vi "Simulation Call Statechart (DLL).vi"(4 "operation":T6, 5 "Robot Index":i32, 8 "error in (no error)":errorcluster, 10 "Array Sensors In":T1[](array[typedef]) {"Kobuki Sensors"."Charger Source" items=["DISCHARGING"=0, "DOCKING_CHARGED"=2, "DOCKING_CHARGING"=6, "ADAPTER_CHARGED"=18, "ADAPTER_CHARGING"=22]; "accelerometer"."z axis (g)" format="%.3f"; "accelerometer"."y axis (g)" format="%.3f"; "accelerometer"."x axis (g)" format="%.3f"}, 11 "simulator":T7={"configuration"={"maxTime"=5.0, "enableVisualization"=TRUE, "Environment Definition"=path "simulation configuration.ini", "Record Location"=path "Simulation Record.xml", "autograde?"=TRUE, "interactive?"=FALSE, "Feedback Mode"=enum."debug navigation", "Robot State Charts"=[path "C:/Users/blueuser/Desktop/Robo Sim Berkley/cpsgrader-release-0.4/Simulators/EECS149lab/src/LabVIEW/statechart/Simulation Statechart.vi"], "statechart"=path "C:/Users/blueuser/Desktop/Robo Sim Berkley/cpsgrader-release-0.4/Simulators/EECS149lab/src/LabVIEW/statechart/Simulation Statechart.vi"}, "Statechart\ndisplay"=refnum, "first step?"=FALSE, "Robots Simulation Statecharts"=[], "Robots"=[]}) -> (0 "error out":errorcluster, 2 "Array Sensors Out":T1[](array[typedef]) {"Kobuki Sensors"."Charger Source" items=["DISCHARGING"=0, "DOCKING_CHARGED"=2, "DOCKING_CHARGING"=6, "ADAPTER_CHARGED"=18, "ADAPTER_CHARGING"=22]; "accelerometer"."z axis (g)" format="%.3f"; "accelerometer"."y axis (g)" format="%.3f"; "accelerometer"."x axis (g)" format="%.3f"}, 3 "simulator":T7={"configuration"={"maxTime"=5.0, "enableVisualization"=TRUE, "Environment Definition"=path "simulation configuration.ini", "Record Location"=path "Simulation Record.xml", "autograde?"=TRUE, "interactive?"=FALSE, "Feedback Mode"=enum."debug navigation", "Robot State Charts"=[path "C:/Users/blueuser/Desktop/Robo Sim Berkley/cpsgrader-release-0.4/Simulators/EECS149lab/src/LabVIEW/statechart/Simulation Statechart.vi"], "statechart"=path "C:/Users/blueuser/Desktop/Robo Sim Berkley/cpsgrader-release-0.4/Simulators/EECS149lab/src/LabVIEW/statechart/Simulation Statechart.vi"}, "Statechart\ndisplay"=refnum, "first step?"=FALSE, "Robots Simulation Statecharts"=[], "Robots"=[]})   [LabVIEW 2015]
uses:
  Simulator.ctl
  CyberSim interface/Simulation Configuration.ctl
  autograder/feedbackMode.ctl
  Multi Bot Code/RobotData.ctl
  <instrlib>/DC Motor Controller/HAIOL/DC Motor Controller.lvclass
  Simulation Call Statechart Operation.ctl
  shared/Sensors.ctl
  shared/Accelerometer.ctl
  Kobuki/KobukiSensors.ctl
  Kobuki/Kobuki Bumps and WheelDrops.ctl
  Kobuki/Kobuki Buttons.ctl
panel:
  # "Electrical: charging, battery, OI mode"
  # "Sensors: bump, cliff, button, wheel drop"
  # "Motors:"
  # "Inertia"
  # "Electrical: charging, battery, OI mode"
  # "Sensors: bump, cliff, button, wheel drop"
  # "Motors:"
  # "Inertia"
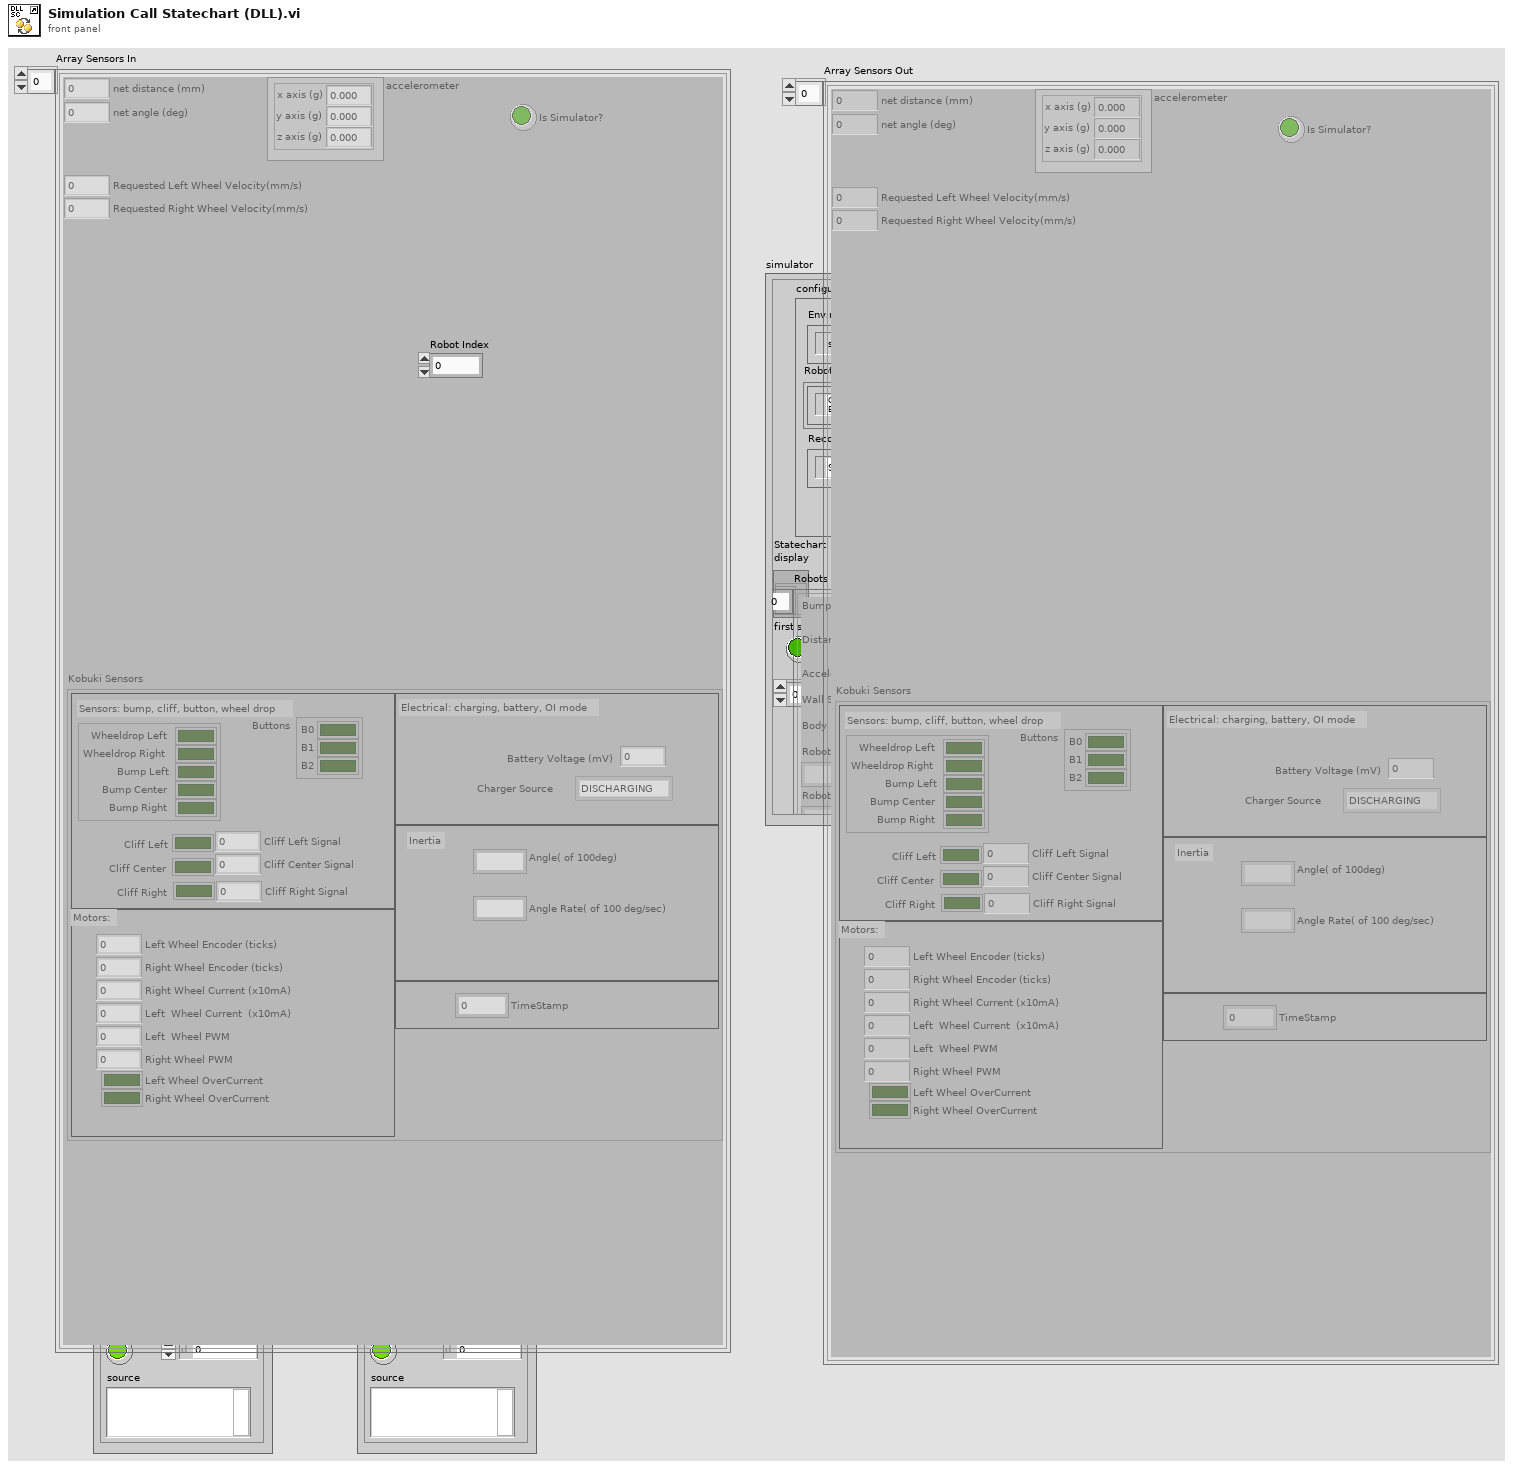
[diagram p1: front panel]
types:
  T1 = typedef "Sensors.ctl" = cluster{"net distance (mm)":i32, "net angle (deg)":i32, "accelerometer":T2, "Is Simulator?":bool, "Kobuki Sensors":T3, "Requested Left Wheel Velocity(mm/s)":i32, "Requested Right Wheel Velocity(mm/s)":i32}
  T2 = typedef "Accelerometer.ctl" = cluster{"x axis (g)":dbl, "y axis (g)":dbl, "z axis (g)":dbl}
  T3 = typedef "KobukiSensors.ctl" = cluster{"Bumps + Wheel Drops":T4, "Cliff Left":bool, "Cliff Center":bool, "Cliff Right":bool, "Cliff Left Signal":u16, "Cliff Center Signal":u16, "Cliff Right Signal":u16, "Buttons":T5, "Left Wheel Encoder (ticks)":u16, "Right Wheel Encoder (ticks) ":u16, "Left  Wheel PWM":i8, "Right Wheel PWM":i8, "Left Wheel OverCurrent":bool, "Right Wheel OverCurrent ":bool, "Right Wheel Current (x10mA)":i16, "Left  Wheel Current  (x10mA)":i16, "TimeStamp":u16, "Battery Voltage (mV)":i16, "Angle( of 100deg)":i16, "Angle Rate( of 100 deg/sec)":i16, "Charger Source ":i8}
  T4 = typedef "Kobuki Bumps and WheelDrops.ctl" = cluster{"Wheeldrop Left":bool, "Wheeldrop Right":bool, "Bump Left":bool, "Bump Center":bool, "Bump Right":bool}
  T5 = typedef "Kobuki Buttons.ctl" = cluster{"B0":bool, "B1":bool, "B2":bool}
  T6 = typedef "Simulation Call Statechart Operation.ctl" = enum16{"Initialize", "Call Statechart", "Finalize"}
  T7 = typedef "Simulator.ctl" = cluster{"configuration":T8, "Statechart\ndisplay":refnum<vi>, "first step?":bool, "Robots Simulation Statecharts":path[], "Robots":T10[]}
  T8 = typedef "Simulation Configuration.ctl" = cluster{"maxTime":sgl, "enableVisualization":bool, "Environment Definition":path, "Record Location":path, "autograde?":bool, "interactive?":bool, "Feedback Mode":T9, "Robot State Charts":path[], "statechart":path}
  T9 = typedef "feedbackMode.ctl" = enum32{"debug navigation", "debug hill climb", "autograde navigation", "autograde hill climb"}
  T10 = typedef "RobotData.ctl" = cluster{"Bump Sensors":refnum<k20>[], "Distance Sensors":refnum<k20>[], "Accelerometer":refnum<k20>, "Wall Sensor":refnum<k20>, "Body":refnum<k20>, "RobotID":string, "RobotType":string, "Left Motor":refnum<class "DC Motor Controller.lvclass">, "Right Motor":refnum<class "DC Motor Controller.lvclass">}
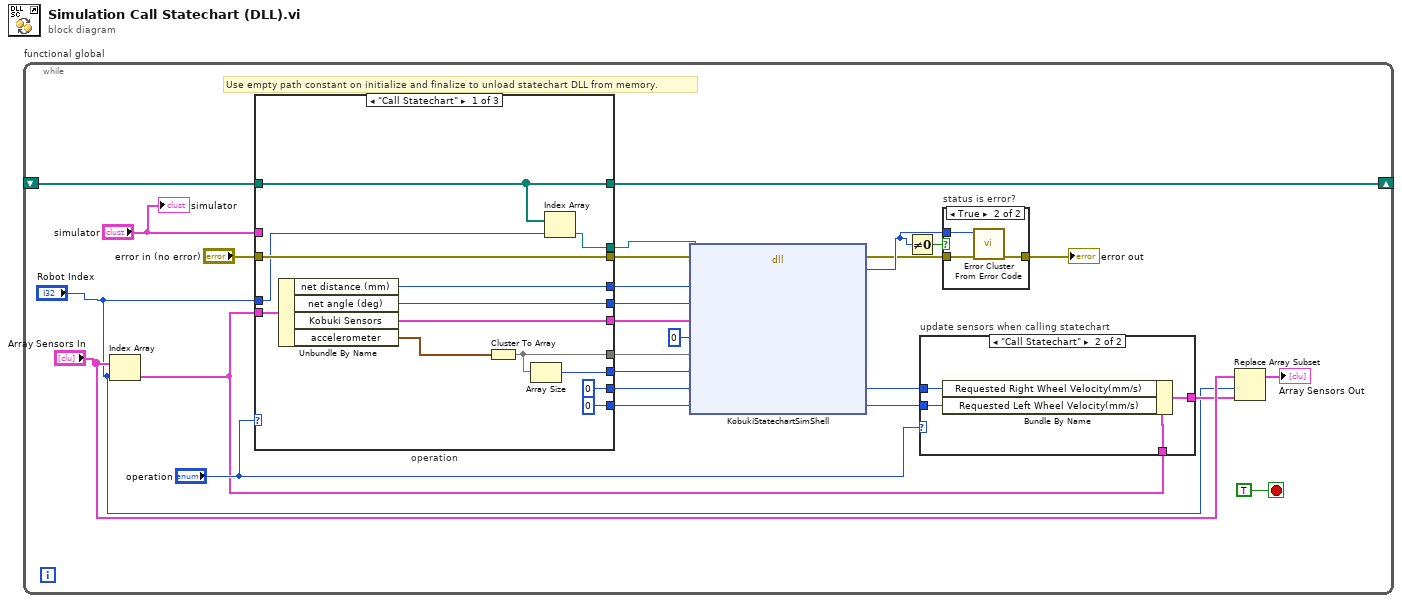
[diagram p0: block diagram]
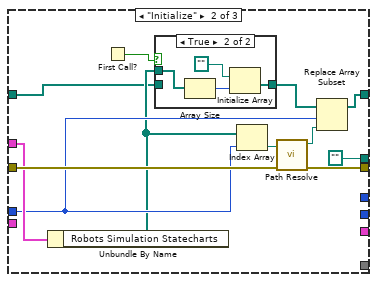
[diagram p4: hidden frame]
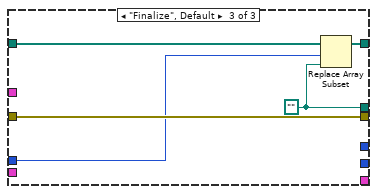
[diagram p6: hidden frame]
diagram:
  n1 = while "functional global" {
    shift-right: [w21] -> _
    shift-left: _ -> [w20]
    stop <- TRUE stop-if-true
    # "Use empty path constant on initialize and finalize to unload statechart DLL from memory."
    n2 = Index Array(array="Array Sensors In", index="Robot Index") -> (element=w19:T1)
    n3 = case "operation" shown="\"Call Statechart\"" "operation" {
      tunnel: "error in (no error)" -> [w49 w61 w71]
      tunnel: [w49 w60 w71] -> w12
      tunnel: [w40 path "" w68] -> w14
      tunnel: [w39 w56 w69] -> w21
      tunnel: w20 -> [w39 w52 w70]
      tunnel: [w47 _ _] -> w11
      tunnel: [w46 _ _] -> w10
      tunnel: [w45 _ _] -> w5
      tunnel: [w44 _ _] -> w4
      tunnel: [i16 0 ("rightWheelSpeed") _ _] -> w3
      tunnel: [i16 0 ("rightWheelSpeed") _ _] -> w2
      tunnel: w19 -> [w41 _ _]
      tunnel: "simulator" -> [_ w58 _]
      tunnel: "Robot Index" -> [w38 w54 w67]
      tunnel: [w37 _ _] -> w13
      frame "Call Statechart" {
        n4 = Unbundle By Name(w41) -> ("net distance (mm)"=w47:i32, "net angle (deg)"=w46:i32, "Kobuki Sensors"=w37:T3, "accelerometer"=w48:T2)
        n5 = Cluster To Array(cluster=w48) -> (array=w45:dbl[])
        n6 = Array Size(array=w45) -> (size(s)=w44:i32)
        n7 = Index Array(array=w39, index=w38) -> (element=w40:path)
      }
      frame "Initialize" {
        n8 = Unbundle By Name(w58) -> ("Robots Simulation Statecharts"=w53:path[])
        n9 = First Call?() -> (First Call?: T/F=w50:bool)
        n10 = case shown="True" w50 {
          tunnel: w52 -> [w62 _]
          tunnel: [w62 w64] -> w51
          tunnel: w53 -> [_ w65]
          frame False {
          }
          frame True {
            n11 = Array Size(array=w65) -> (size(s)=w66:i32)
            n12 = Initialize Array(path "", w66) -> (w64:path[])
          }
        }
        n13 = Index Array(array=w53, index=w54) -> (element=w57:path)
        n14 = call "Path Resolve.vi"("Error In"=w61, "absolute or relative path"=w57) -> ("Error Out"=w60:errorcluster, "resolved path"=w55:path)  [unwired: 8 in]
        n15 = Replace Array Subset(array=w51, new element=w55, index=w54) -> (w56:path[])
      }
      frame "Finalize", Default {
        w68 = path ""
        n16 = Replace Array Subset(array=w70, new element=w68, index=w67) -> (w69:path[])
      }
    }
    n17 = dll-call lib="D:/Users/jjensen/workspace/Simulated iRobot Navigation/Release/libSimulated iRobot Navigation.dll" fn="KobukiStatechartSimShell"(path in=w14, error in=w12, "netDistance"=w11, "netAngle"=w10, "sensors"=w13, "sensorStreamSize"=0, "accelAxes"=w5, "accelAxesSize"=w4, "rightWheelSpeed"=w3, "leftWheelSpeed"=w2) -> (error out=w6:errorcluster, "status"=w9:i32, "rightWheelSpeed"=w8:i16, "leftWheelSpeed"=w7:i16)  [unwired: 7 in, 1 out]
    n18 = Not Equal To 0?(x=w9) -> (x != 0?=w25:bool)
    n19 = case "update sensors when calling statechart" shown="\"Call Statechart\"" "operation" {
      tunnel: w8 -> [_ w32]
      tunnel: w7 -> [_ w31]
      tunnel: w19 -> [w28 w30]
      tunnel: [w28 w29] -> w17
      frame Default {
      }
      frame "Call Statechart" {
        n20 = Bundle By Name(cluster=w30, "Requested Right Wheel Velocity(mm/s)"=w32, "Requested Left Wheel Velocity(mm/s)"=w31) -> (w29:T1)
      }
    }
    n21 = case "status is error?" shown="True" w25 {
      tunnel: w9 -> [_ w36]
      tunnel: w6 -> [w33 w35]
      tunnel: [w33 w34] -> w24
      frame False {
      }
      frame True {
        n22 = call <vilib>:"Error Cluster From Error Code.vi"("error in (no error)"=w35, "error code (0)"=w36) -> ("error out"=w34:errorcluster)  [unwired: 7 in]
      }
    }
    "error out" <- w24
    n23 = Replace Array Subset(array="Array Sensors In", new element=w17, index="Robot Index") -> (→"Array Sensors Out":T1[])
    "simulator" <- "simulator"
  }
